vi "Create WebSocket Resource.vi"(7 "Manager Type":refnum<class "WebSocket Manager.lvclass">, 8 "error in (no error)":errorcluster, 10 "Path":string, 11 "Server in":refnum<class "Server.lvclass">) -> (0 "error out":errorcluster, 2 "Manager":refnum<class "WebSocket Manager.lvclass">, 3 "Server out":refnum<class "Server.lvclass">)   [LabVIEW 2020, in "HTTP Server.lvlib" / "Server.lvclass"]
doc: "Creates a WebSocket server that responds to websocket upgrade requests at the specified path. Unlike controller paths, WS paths are not specified as a regular expression and must match the entire path exactly. The WS Server that is returned can be registered as an endpoint with messaging or used directly to perform lower latency, bi-directional communication with client-side code (javascript)."
uses:
  Server.lvclass
  Server.lvclass/Server.ctl
  WebSocket Manager/WebSocket Manager.lvclass
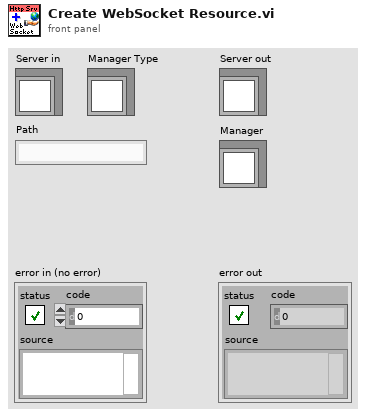
[diagram p1: front panel]
types:
  T1 = typedef "HTTP Server.lvlib/WebSocket Data.ctl" = cluster{"WS Managers":map{string, refnum<class "WebSocket Manager.lvclass">}}
  T2 = map{string, refnum<class "WebSocket Manager.lvclass">}
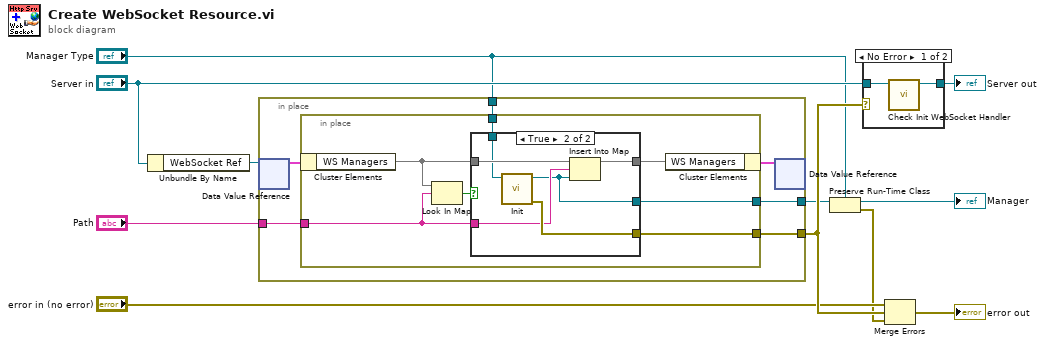
[diagram p0: block diagram]
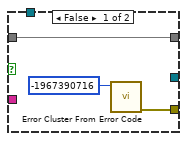
[diagram p2: hidden frame]
diagram:
  n1 = Unbundle By Name("Server in") -> ("WebSocket Ref"=w9:refnum<data-value>)
  n2 = in-place {
    in-place-border: "Path" -> [w15]
    in-place-border: [w14] -> w11
    in-place-border: "Manager Type" -> [w13]
    in-place-border: [w12] -> w4
    n3 = in-place-dvr #1(w9) -> (w17:T1)  [unwired: 1 out]
    n4 = in-place {
      in-place-border: w15 -> [w23]
      in-place-border: [w20] -> w14
      in-place-border: w13 -> [w19]
      in-place-border: [w18] -> w12
      n5 = in-place-cluster #2(w17) -> ("WS Managers"=w22:T2)
      n6 = Look In Map(map=w22, key=w23) -> (key not found?=w24:bool)  [unwired: 1 in, 1 out]
      n7 = case shown="True" w24 {
        tunnel: w23 -> [_ w31]
        tunnel: w22 -> [w27 w32]
        tunnel: [w27 w30] -> w21
        tunnel: [w25 w33] -> w20
        tunnel: w19 -> [_ w29]
        tunnel: [_ w28] -> w18
        frame False {
          n8 = call <vilib>:"Error Cluster From Error Code.vi"("error code (0)"=-1967390716) -> ("error out"=w25:errorcluster)  [unwired: 8 in]
        }
        frame True {
          n9 = call "Init.vi"("WebSocket Manager in"=w29) -> ("error out"=w33:errorcluster, "WebSocket Manager out"=w28:refnum<class "WebSocket Manager.lvclass">)  [unwired: 9 in]
          n10 = Insert Into Map(map in=w32, key=w31, value=w28) -> (map out=w30:T2)  [unwired: 2 out]
        }
      }
      n11 = in-place-cluster #2("WS Managers"=w21) -> (w16:T1)
    }
    n12 = in-place-dvr #1(w16) -> ()  [unwired: 2 out]
  }
  n13 = Preserve Run-Time Class(object in=w4, 2:"Manager Type") -> (object out=→"Manager":refnum<class "WebSocket Manager.lvclass">, error out=w2:errorcluster)  [unwired: 1 in]
  n14 = case shown="No Error" w11 {
    tunnel: "Server in" -> [w35 w36]
    tunnel: [w34 w36] -> w5
    frame No Error {
      n15 = call "Check Init WebSocket Handler.vi"("Server in"=w35) -> ("Server out"=w34:refnum<class "Server.lvclass">)  [unwired: 9 in, 1 out]
    }
    frame Error {
    }
  }
  "Server out" <- w5
  n16 = Merge Errors("error in (no error)", w11, w2) -> (→"error out":errorcluster)
